vi "MasterAccelerometerSample3.vi"   [LabVIEW 2018]
uses:
  DataTypes/AccelerometerRecord3.ctl
  <vilib>/rvi/Emulation/niFpgaGetClockAttributes.vi
  <vilib>/rvi/Emulation/niFpgaSctlEmulationGetInTimedLoop.vi
  <vilib>/rvi/Emulation/niFpgaEmulationReportErrorSimple.vi
  <vilib>/rvi/Emulation/niFpgaEmulationIsFPGAContextNoSignature.vi
  <vilib>/rvi/DataTransferAndStorage/Container/Common/niFpgaContainerGetUniqueNameForEmu.vi
  <vilib>/rvi/Memory/Memory_Emulation/niFpgaMemoryEmulationCacheClearOnFirstRun.vi
  <vilib>/rvi/Memory/Memory_Emulation/nirvimemoryEmulationManagerCache_MakeExclusive.vi
  <vilib>/rvi/Memory/Memory_Emulation/niFpgaMemoryEmulationValidateCache.vi
  <vilib>/rvi/Memory/Memory_Emulation/nirvimemoryEmulationManagerCache_InsertValue.vi
  <vilib>/Utility/error.llb/Clear Errors.vi
  <vilib>/rvi/Memory/Memory_Emulation/nirvimemoryEmulationManagerCache_ReleaseExclusive.vi
  <vilib>/rvi/Memory/Memory_Emulation/nirvimemoryEmulationManagerCache_GetValue.vi
  <vilib>/rvi/Memory/Memory_Emulation/nirvimemoryEmulationManagerCache_SetValue.vi
  <vilib>/rvi/Emulation/niFpgaProcessEmulError.vi
  <vilib>/rvi/eio/common/nirviEmuTemplateMethod_errors.vi
  <vilib>/rvi/errors/niFpgaSetErrorForExecOnDevCompSimple.vi
  <vilib>/rvi/eio/common/nirviEmuReportErrorAndStop.vi
  <vilib>/rvi/FIFO/Fifo_Resource/nirvififoEmulationSetSize.vi
  <vilib>/rvi/FIFO/Fifo_Resource/nirviFifoEmulationQueueMgr.vi
  <instcachedir>/0/nirviFifoEmulationQueueMgr_E5CAEC123FF24DC58D834DCA3CDAA9B5.lvgen/nirviFifoEmulationQueueMgr_E5CAEC123FF24DC58D834DCA3CDAA9B5_033.vi
  <vilib>/rvi/FIFO/Fifo_Resource/nirvififoEmulationDetermineInputValidOut.vi
  <vilib>/rvi/FIFO/Fifo_Resource/nirvififoEmulationCreateLock.vi
  <vilib>/rvi/FIFO/Fifo_Resource/nirvififoEmulationObtainLock.vi
  <vilib>/rvi/FIFO/Fifo_Resource/nirvififoEmulationReleaseLock.vi
  <vilib>/rvi/occurrence/nirviWaitOnOccurrenceBase.vi
  <vilib>/rvi/errors/nirviReportUnexpectedCaseInternalError.vi
  <vilib>/rvi/errors/nirviReportUnexpectedCaseInternalError (U32).vi
  <vilib>/rvi/Emulation/niFpgaCriticalErrorInLSC.vi
  <vilib>/rvi/DataTransferAndStorage/Container/XNode/niFpgaContainer.xnode
  <vilib>/rvi/DataTransferAndStorage/Register/Emulation/niFpgaRegisterEmulation.vi
  <vilib>/eio/EIOMethodNode/EIOMethodNode.xnode
  <vilib>/eio/EIONode/EIONode.xnode
  <vilib>/rvi/FIFO/Fifo_Resource/nirvififoEmulationWrite.vi
types:
  T1 = typedef "AccelerometerRecord3.ctl" = cluster{"Timestamp":u64, "Accelerometers":sgl[]}
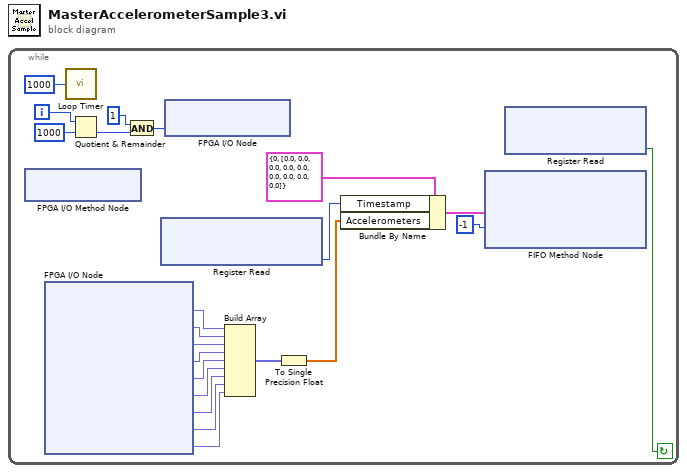
[diagram p0: block diagram]
diagram:
  n1 = while {
    i -> [w2]
    stop <- w3 continue-if-true
    n2 = xnode "FPGA I/O Method Node"() -> ()  [unwired: 1 in, 1 out]
    n3 = xnode "FPGA I/O Node"() -> ("Accelerometer1/AI0"=w20:fxp<+/-,24,4>, "Accelerometer1/AI1"=w19:fxp<+/-,24,4>, "Accelerometer1/AI2"=w18:fxp<+/-,24,4>, "Accelerometer2/AI0"=w17:fxp<+/-,24,4>, "Accelerometer2/AI1"=w16:fxp<+/-,24,4>, "Accelerometer2/AI2"=w15:fxp<+/-,24,4>, "Accelerometer3/AI0"=w14:fxp<+/-,24,4>, "Accelerometer3/AI1"=w13:fxp<+/-,24,4>, "Accelerometer3/AI2"=w12:fxp<+/-,24,4>)  [unwired: 9 in, 9 out]
    n4 = call "Loop Timer"("Count(uSec)"=u32 1000 ("Data")) -> ()  [unwired: 1 out]
    n5 = Quotient & Remainder(x=w2, y=i16 1000) -> (floor(x/y)=w7:i32)  [unwired: 1 out]
    n6 = And(x=1 ("y"), y=w7) -> (x .and. y?=w5:i32)
    n7 = xnode ("Register Read")() -> ("Data"=w9:u64)  [unwired: 1 in, 1 out]
    n8 = xnode "FPGA I/O Node"("USER FPGA LED"=w5) -> ()  [unwired: 1 in, 1 out]
    n9 = Build Array(w20, w19, w18, w17, w16, w15, w14, w13, w12) -> (w21:fxp<+/-,24,4>[])
    n10 = To Single Precision Float(number=w21) -> (single precision float=w10:sgl[])
    n11 = Bundle By Name(cluster=T1 {"Timestamp"=0, "Accelerometers"=[0.0, 0.0, 0.0, 0.0, 0.0, 0.0, 0.0, 0.0, 0.0]} ("AccelerometerSample3"), "Timestamp"=w9, "Accelerometers"=w10) -> (w1:T1)
    n12 = xnode ("FIFO Method Node")("Element"=w1, "Timeout"=-1) -> ()  [unwired: 1 in, 2 out]
    n13 = xnode ("Register Read")() -> ("Data"=w3:bool)  [unwired: 1 in, 1 out]
  }
